vi "Trial v1.vi"(2 "error in (no error)":errorcluster, 3 "queue in":refnum<queue>, 4 "DDA":bool=TRUE) -> (0 "error out":errorcluster, 1 "queue out":refnum<queue>)   [LabVIEW 2017]
uses:
  SubVI/Global.vi
  <vilib>/Analysis/NI_AALPro.lvlib
  <vilib>/robotics/Kinematics/NI_Kinematics.lvlib
  Control/RPY.ctl
  Control/Damping.ctl
  <vilib>/Analysis/NI_AALBase.lvlib
  <vilib>/Analysis/baseanly.llb/Real Dot Product.vi
  <vilib>/Analysis/_algsub.llb/Real Vector Norm.vi
panel:
  out "R":dbl
  out "Rbar":dbl
  out "delta":dbl
  in  "Algorithm Parameter":T1={"lambda w"=0.0, "lambda theta"=0.0, "alpha w"=0.0, "alpha theta"=0.0, "alpha Rbar"=0.1}
  in  "n":i32=3
  in  "Reward Parameter":cluster{"C":dbl, "alpha":dbl}={"C"=100.0, "alpha"=1.0}
  in  "lower limit (RoM)":dbl=15.0
  in  "upper limit (RoM)":dbl=85.0
  in  "Time Target (s)":dbl=1.0
  in  "epsilon":dbl=0.1
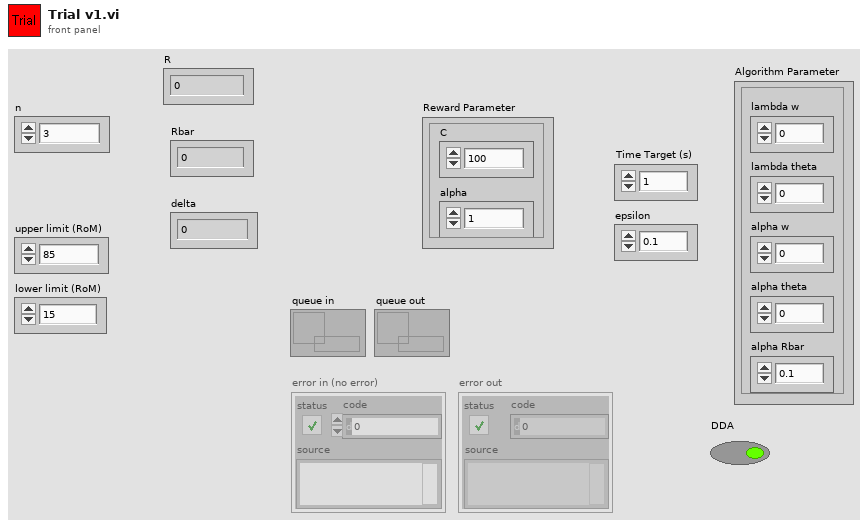
[diagram p1: front panel]
types:
  T1 = cluster{"lambda w":dbl, "lambda theta":dbl, "alpha w":dbl, "alpha theta":dbl, "alpha Rbar":dbl}
  T2 = typedef "Damping.ctl" = cluster{"Cx":dbl, "Cy":dbl, "Cz":dbl}
  T3 = typedef "RPY.ctl" = cluster{"roll":dbl, "pitch":dbl, "yaw":dbl}
  T4 = typedef "NI_Matrix.lvlib/RealMatrix.ctl" = dbl[][]
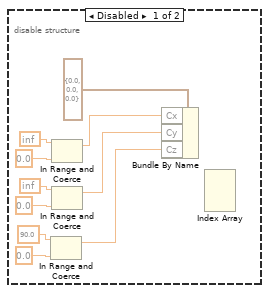
[diagram p2: hidden frame]
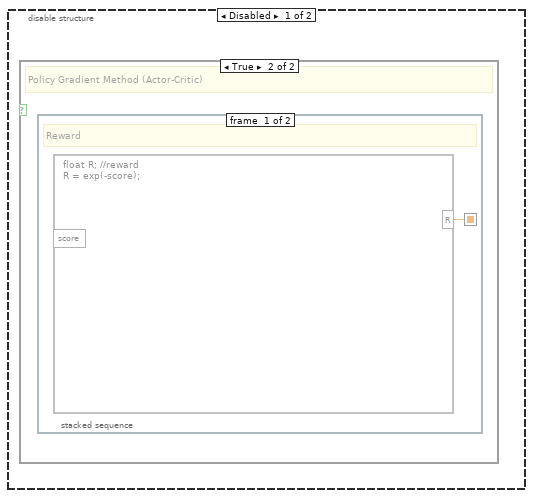
[diagram p3: hidden frame]
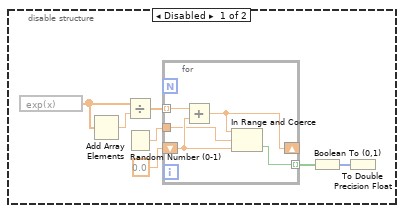
[diagram p6: hidden frame]
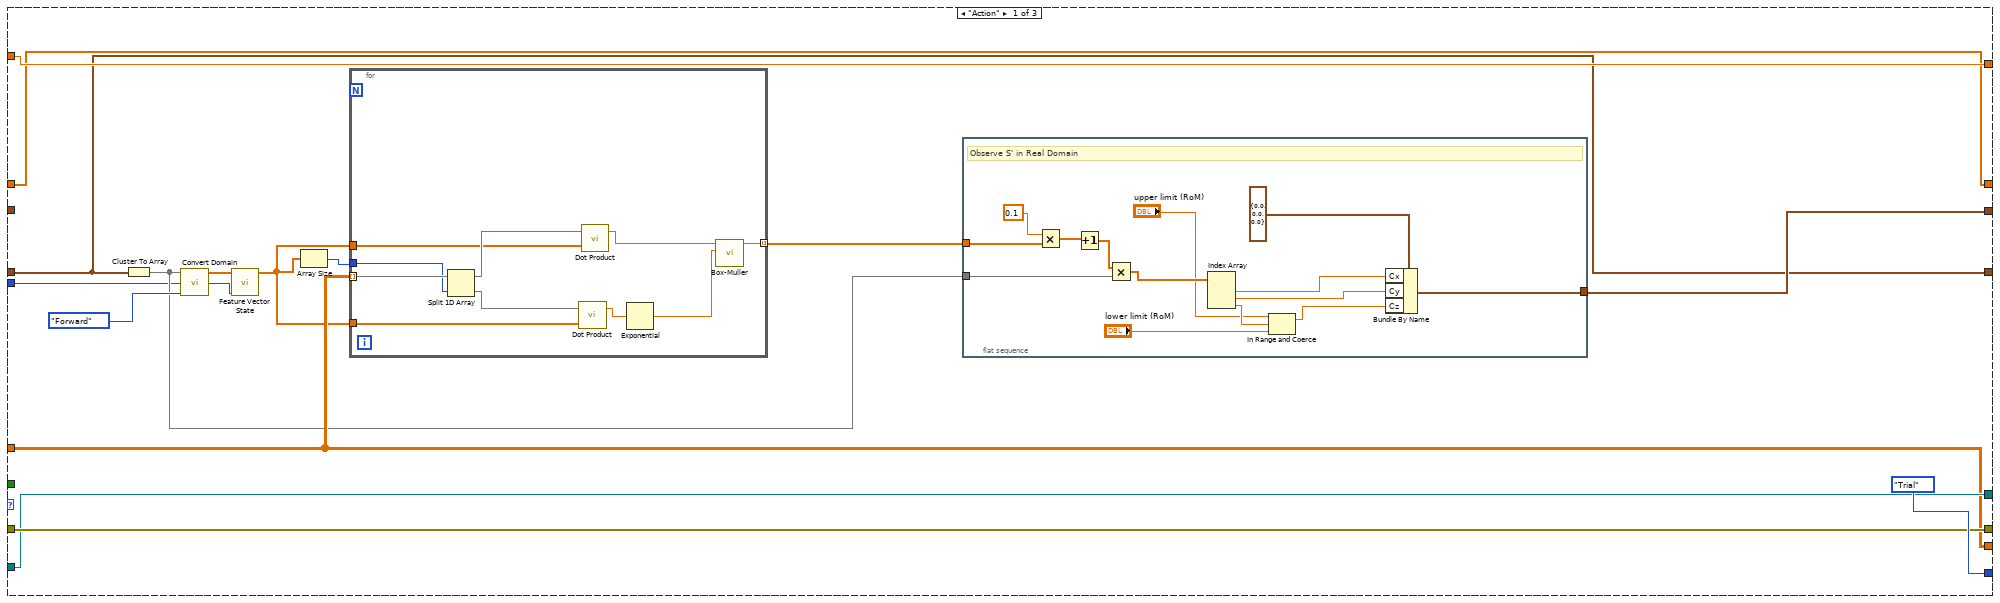
[diagram p7: hidden frame]
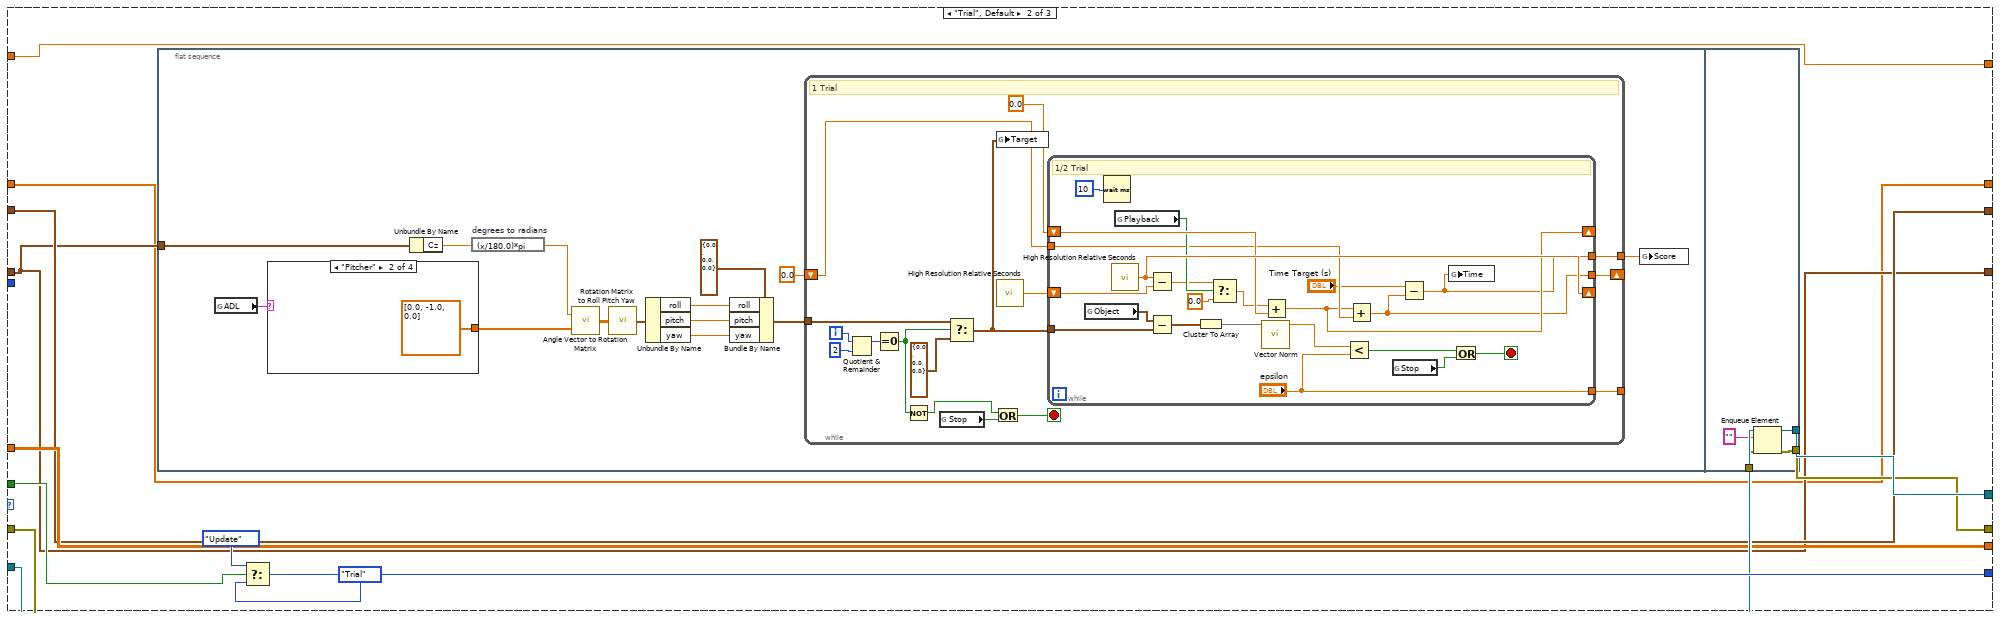
[diagram p8: hidden frame]
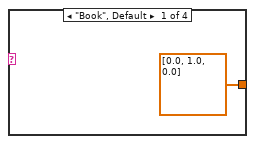
[diagram p9: hidden frame]
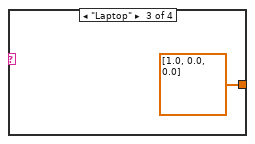
[diagram p10: hidden frame]
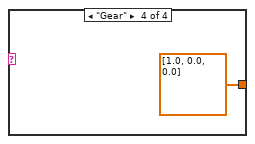
[diagram p11: hidden frame]
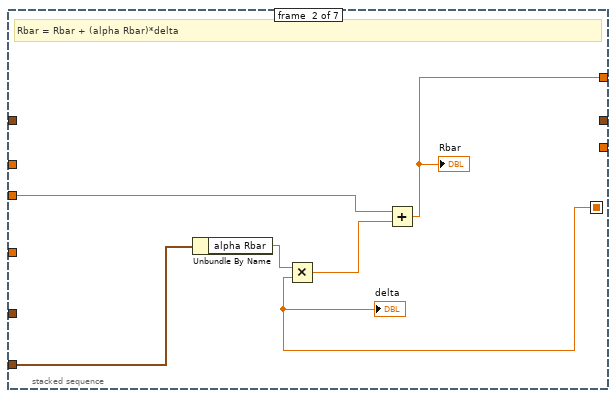
[diagram p12: hidden frame]
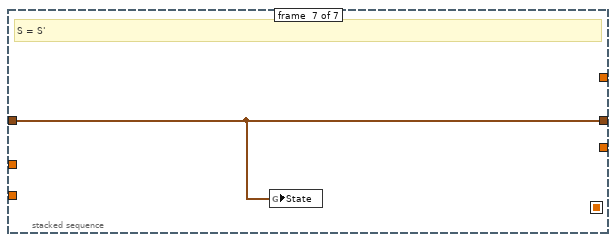
[diagram p17: hidden frame]
diagram:
  n1 = flat-sequence {
    tunnel: "error in (no error)" -> [w17]
    tunnel: "queue in" -> [w19]
    tunnel: "DDA" -> [w12]
    tunnel: [w18] -> w2
    tunnel: [w16] -> w1
    frame #0 {
      n2 = flat-sequence {
        tunnel: ["n"] -> w11
        tunnel: [w29] -> w10
        tunnel: [w28] -> w9
        tunnel: [w28] -> w8
        tunnel: [w26] -> w7
        tunnel: [w20] -> w6
        frame #0 {
          w29 = 0.0  # Rbar
          w22 = 0.0 ("element")
          w25 = dbl[] [0.0, 0.0, 0.0] ("array")
          n3 = call "Feature Vector State.vi"("n x(s)"="n", "state"=w25) -> ("x(s)"=w35:dbl[])  [unwired: 9 in]
          n4 = call "Feature Vector State.vi"("n x(s)"="n", "state"=w25) -> ("x(s)"=w33:dbl[])  [unwired: 9 in]
          n5 = call "Feature Vector State.vi"("n x(s)"="n", "state"=w25) -> ("x(s)"=w24:dbl[])  [unwired: 9 in]
          n6 = Array Size(array=w24) -> (size(s)=w23:i32)
          n7 = Array Size(array=w35) -> (size(s)=w34:i32)
          n8 = Array Size(array=w33) -> (size(s)=w32:i32)
          n9 = Initialize Array(w22, w23) -> (w20:dbl[])
          n10 = Initialize Array(w22, w34) -> (w31:dbl[])
          n11 = Initialize Array(w22, w32) -> (w30:dbl[])
          n12 = global read "Global.vi" "State"() -> (w28:T2)
          n13 = Build Array (concatenate)(w31, w30) -> (w27:dbl[])
          n14 = Build Array(w27, w27, w27) -> (w26:dbl[][])
        }
      }
      n15 = Select(t=enum16{"Action", "Trial", "Update"}."Action", s=w12, f=enum16{"Action", "Trial", "Update"}."Trial") -> (s? t:f=w13:enum16{"Action", "Trial", "Update"})
      n16 = while {
        shift-right: [w48] -> w18
        shift-left: w19 -> [w50]
        shift-right: [w47] -> w16
        shift-left: w17 -> [w49]
        shift-right: [w52] -> _
        shift-left: w13 -> [w53]
        tunnel: w12 -> [w51]
        tunnel: w11 -> [w46]
        shift-right: [w45] -> _
        shift-left: w7 -> [w44]
        shift-right: [w42] -> _
        shift-left: w10 -> [w43]
        shift-right: [w38] -> _
        shift-left: w9 -> [w40]
        shift-right: [w41] -> _
        shift-left: w8 -> [w39]
        shift-right: [w36] -> _
        shift-left: w6 -> [w37]
        stop <- w54 stop-if-true
        # "State Machine"
        n17 = case shown="\"Update\"" w53 {
          tunnel: [enum16{"Action", "Trial", "Update"}."Trial" w104 enum16{"Action", "Trial", "Update"}."Action"] -> w52
          tunnel: w51 -> [_ w106 _]
          tunnel: w50 -> [w65 w103 w182]
          tunnel: w49 -> [w66 w102 w183]
          tunnel: [w65 w101 w182] -> w48
          tunnel: [w66 w100 w183] -> w47
          tunnel: w46 -> [w57 _ w173]
          tunnel: [w64 w98 w184] -> w45
          tunnel: w44 -> [w64 w98 w184]
          tunnel: w43 -> [w60 w97 w175]
          tunnel: [w60 w97 w169] -> w42
          tunnel: w40 -> [w58 w95 w172]
          tunnel: [w59 w96 w171] -> w41
          tunnel: w39 -> [_ w96 w177]
          tunnel: [w58 w95 w171] -> w38
          tunnel: w37 -> [w55 w94 w174]
          tunnel: [w55 w94 w168] -> w36
          frame "Action" {
            n18 = Cluster To Array(cluster=w58) -> (array=w61:dbl[])
            n19 = call "Convert Domain.vi"("Direction"=enum16{"Forward", "Backward"}."Forward", "Real"=w61) -> ("Unit"=w67:dbl[])  [unwired: 9 in]
            n20 = call "Feature Vector State.vi"("n x(s)"=w57, "state"=w67) -> ("x(s)"=w56:dbl[])  [unwired: 9 in]
            n21 = Array Size(array=w56) -> (size(s)=w63:i32)
            n22 = for {
              tunnel: w64 -> [w93] mode=indexing
              tunnel: w56 -> [w90]
              tunnel: w56 -> [w89]
              tunnel: [w85] -> w62 mode=indexing
              tunnel: w63 -> [w84]
              n23 = Split 1D Array(array=w93, index=w84) -> (first subarray=w92:dbl[], second subarray=w91:dbl[])
              n24 = call-poly <vilib>:"Dot Product.vi"("Y Vector"=w89, "X Vector"=w91) -> ("X * Y"=w88:dbl)  [unwired: 1 out]
              n25 = call-poly <vilib>:"Dot Product.vi"("Y Vector"=w90, "X Vector"=w92) -> ("X * Y"=w87:dbl)  [unwired: 1 out]
              n26 = Exponential(1:w88) -> (0:w86:dbl)
              n27 = call "Box-Muller.vi"("sigma"=w86, "mu"=w87) -> ("x"=w85:dbl)  [unwired: 9 in]
            }
            n28 = flat-sequence {
              tunnel: w62 -> [w83]
              tunnel: w61 -> [w79]
              tunnel: [w70] -> w59
              frame #0 {
                # "Observe S' in Real Domain"
                n29 = Multiply(x=0.1, y=w83) -> (x*y=w81:dbl[])
                n30 = Increment(x=w81) -> (x+1=w80:dbl[])
                n31 = Multiply(x=w80, y=w79) -> (x*y=w75:dbl[])
                n32 = Index Array(array=w75) -> (element #1=w77:dbl, element #2=w76:dbl, element #3=w74:dbl)  [unwired: 3 in]
                n33 = In Range and Coerce(upper limit="upper limit (RoM)", x=w74, lower limit="lower limit (RoM)") -> (coerced(x)=w73:dbl)  [unwired: 1 out]
                n34 = Bundle By Name(cluster=T2 {"Cx"=0.0, "Cy"=0.0, "Cz"=0.0} ("State"), "Cx"=w77, "Cy"=w76, "Cz"=w73) -> (w70:T2)
              }
            }
          }
          frame "Trial", Default {
            n35 = flat-sequence {
              tunnel: w95 -> [w107]
              tunnel: w103 -> [w167]
              tunnel: w102 -> [w166]
              tunnel: [w165] -> w101
              tunnel: [w164] -> w100
              frame #0 {
                n36 = global read "Global.vi" "ADL"() -> (w111:string)
                n37 = case shown="\"Pitcher\"" w111 {
                  tunnel: [dbl[] [0.0, 1.0, 0.0] dbl[] [0.0, -1.0, 0.0] dbl[] [1.0, 0.0, 0.0] dbl[] [1.0, 0.0, 0.0]] -> w110
                  frame "Book", Default {
                  }
                  frame "Pitcher" {
                  }
                  frame "Laptop" {
                  }
                  frame "Gear" {
                  }
                }
                n38 = Unbundle By Name(w107) -> ("Cz"=w109:dbl)
                n39 = expression code="(x/180.0)*pi" "degrees to radians"(w109) -> (w112:dbl)
                n40 = call <vilib>:"Angle Vector to Rotation Matrix.vi"("vector"=w110, "angle"=w112) -> ("rotation matrix"=w115:T4)
                n41 = call <vilib>:"Rotation Matrix to Roll Pitch Yaw.vi"("rotation matrix"=w115) -> ("angles"=w116:cluster{"roll":dbl, "pitch":dbl, "yaw":dbl})
                n42 = Unbundle By Name(w116) -> ("roll"=w117:dbl, "pitch"=w118:dbl, "yaw"=w119:dbl)
                n43 = Bundle By Name(cluster=T3 {"roll"=0.0, "pitch"=0.0, "yaw"=0.0} ("Target"), "roll"=w117, "pitch"=w118, "yaw"=w119) -> (w113:T3)
                n44 = while {
                  tunnel: w113 -> [w135]
                  shift-right: [w127] -> _
                  shift-left: 0.0 -> [w128]
                  tunnel: [w126] -> _
                  tunnel: [w125] -> w108
                  i -> [w138]
                  stop <- w131 stop-if-true
                  # "1 Trial"
                  n45 = Quotient & Remainder(x=w138, y=2) -> (x-y*floor(x/y)=w136:i32)  [unwired: 1 out]
                  n46 = Equal To 0?(x=w136) -> (x = 0?=w130:bool)
                  n47 = Not(x=w130) -> (.not. x?=w129:bool)
                  n48 = global read "Global.vi" "Stop"() -> (w132:bool)
                  n49 = Select(t=w135, s=w130, f=T3 {"roll"=0.0, "pitch"=0.0, "yaw"=0.0} ("Target")) -> (s? t:f=w133:T3)
                  n50 = Or(x=w129, y=w132) -> (x .or. y?=w131:bool)
                  n51 = global write "Global.vi" "Target"(w133) -> ()
                  n52 = call <vilib>:"High Resolution Relative Seconds.vi"() -> ("relative seconds"=w140:dbl)
                  n53 = while {
                    tunnel: w133 -> [w147]
                    shift-right: [w153] -> _
                    shift-left: w140 -> [w154]
                    shift-right: [w145] -> _
                    shift-left: 0.0 -> [w152]
                    tunnel: w128 -> [w146]
                    tunnel: [w143] -> w127
                    tunnel: ["epsilon"] -> w126
                    tunnel: [w141] -> w125
                    stop <- w155 stop-if-true
                    # "1/2 Trial"
                    n54 = global read "Global.vi" "Object"() -> (w160:T3)
                    n55 = Wait (ms)(milliseconds to wait=u32 10) -> ()  [unwired: 1 out]
                    n56 = call <vilib>:"High Resolution Relative Seconds.vi"() -> ("relative seconds"=w153:dbl)
                    n57 = global read "Global.vi" "Playback"() -> (w151:bool)
                    n58 = Subtract(x=w153, y=w154) -> (x-y=w150:dbl)
                    n59 = Subtract(x=w160, y=w147) -> (x-y=w161:T3)
                    n60 = Cluster To Array(cluster=w161) -> (array=w162:dbl[])
                    n61 = Select(t=w150, s=w151, f=0.0) -> (s? t:f=w149:dbl)
                    n62 = call-poly <vilib>:"Vector Norm.vi"("Input Vector"=w162) -> ("norm"=w159:dbl)  [unwired: 9 in, 1 out]
                    n63 = Add(x=w149, y=w152) -> (x+y=w145:dbl)
                    n64 = Less?(x=w159, y="epsilon") -> (x < y?=w158:bool)
                    n65 = Add(x=w145, y=w146) -> (x+y=w143:dbl)
                    n66 = global read "Global.vi" "Stop"() -> (w157:bool)
                    n67 = Subtract(x="Time Target (s)", y=w143) -> (x-y=w141:dbl)
                    n68 = global write "Global.vi" "Time"(w141) -> ()
                    n69 = Or(x=w158, y=w157) -> (x .or. y?=w155:bool)
                  }
                }
                n70 = global write "Global.vi" "Score"(w108) -> ()
              }
              frame #1 {
                n71 = Enqueue Element(queue=w167, element="", error in (no error)=w166) -> (queue out=w165:refnum<queue>, error out=w164:errorcluster)  [unwired: 1 in, 1 out]
              }
            }
            n72 = Select(t=enum16{"Action", "Trial", "Update"}."Update", s=w106, f=enum16{"Action", "Trial", "Update"}."Trial") -> (s? t:f=w104:enum16{"Action", "Trial", "Update"})
          }
          frame "Update" {
            n73 = Unbundle By Name("Reward Parameter") -> ("C"=w179:dbl, "alpha"=w178:dbl)
            n74 = global read "Global.vi" "Score"() -> (w181:dbl)
            n75 = formula code="float R = C*exp(-alpha*abs(score));"("score"=w181, "C"=w179, "alpha"=w178) -> ("R"=w176:dbl)
            n76 = stacked-sequence {
              seq-local: [w186 _ _ _ _ _ _] -> [_ w202 _ _ _ _ _]
              tunnel: [_ _ _ _ _ _ w207] -> w171
              tunnel: w177 -> [w195 _ _ _ _ _ w207]
              tunnel: w176 -> [w199 _ _ _ _ _ _]
              tunnel: w175 -> [w198 w205 _ _ _ _ _]
              tunnel: w174 -> [w196 _ _ _ w206 _ _]
              tunnel: w173 -> [w189 _ _ _ _ _ _]
              tunnel: w172 -> [w194 _ _ _ _ _ _]
              tunnel: "Algorithm Parameter" -> [_ w204 _ _ _ _ _]
              tunnel: [_ w200 _ _ _ _ _] -> w169
              tunnel: [_ _ _ _ w206 _ _] -> w168
              frame #0 {
                # "delta = R - Rbar + vhat(S', w) - vhat(S,w)"
                n77 = Subtract(x=w195, y=w194) -> (x-y=w193:T2)
                n78 = Cluster To Array(cluster=w193) -> (array=w192:dbl[])
                n79 = Subtract(x=w199, y=w198) -> (x-y=w197:dbl)
                n80 = call "Convert Domain.vi"("Direction"=enum16{"Forward", "Backward"}."Forward", "Real"=w192) -> ("Unit"=w190:dbl[])  [unwired: 9 in]
                n81 = call "Feature Vector State.vi"("n x(s)"=w189, "state"=w190) -> ("x(s)"=w188:dbl[])  [unwired: 9 in]
                n82 = call-poly <vilib>:"Dot Product.vi"("Y Vector"=w188, "X Vector"=w196) -> ("X * Y"=w187:dbl)  [unwired: 1 out]
                n83 = Add(x=w197, y=w187) -> (x+y=w186:dbl)
                "R" <- w199
              }
              frame #1 {
                # "Rbar = Rbar + (alpha Rbar)*delta"
                n84 = Unbundle By Name(w204) -> ("alpha Rbar"=w203:dbl)
                n85 = Multiply(x=w203, y=w202) -> (x*y=w201:dbl)
                n86 = Add(x=w205, y=w201) -> (x+y=w200:dbl)
                "Rbar" <- w200
                "delta" <- w202
              }
              frame #2 {
                # "zw = (lamda w)*zw + del vhat(S, w)"
              }
              frame #3 {
                # "ztheta = (lambda theta)*ztheta + del ln(pi(A| S, theta))"
              }
              frame #4 {
                # "w = w + (alpha w)*delta*zw"
              }
              frame #5 {
                # "theta = theta + (alpha theta)*delta*ztheta"
              }
              frame #6 {
                # "S = S'"
                n87 = global write "Global.vi" "State"(w207) -> ()
              }
            }
          }
        }
        n88 = global read "Global.vi" "Stop"() -> (w54:bool)
      }
    }
  }
  n89 = disable-structure shown="Enabled" {
    frame Disabled {
      n90 = In Range and Coerce(upper limit=90.0, lower limit=0.0) -> (coerced(x)=w217:dbl)  [unwired: 1 in, 1 out]
      n91 = In Range and Coerce(upper limit=inf, lower limit=0.0) -> (coerced(x)=w215:dbl)  [unwired: 1 in, 1 out]
      n92 = In Range and Coerce(upper limit=inf, lower limit=0.0) -> (coerced(x)=w216:dbl)  [unwired: 1 in, 1 out]
      n93 = Bundle By Name(cluster=T2 {"Cx"=0.0, "Cy"=0.0, "Cz"=0.0} ("State"), "Cx"=w215, "Cy"=w216, "Cz"=w217) -> ()  [unwired: 1 out]
      n94 = Index Array() -> ()  [unwired: 4 in, 3 out]
    }
    frame Enabled {
    }
  }
  n95 = disable-structure shown="Enabled" {
    frame Disabled {
      n96 = expression code="exp(x)"() -> (w220:dbl[])  [unwired: 1 in]
      n97 = Add Array Elements(numeric array=w220) -> (sum=w221:dbl)
      n98 = Divide(x=w220, y=w221) -> (x/y=w218:dbl[])
      n99 = Random Number (0-1)() -> (number: 0 to 1=w222:dbl)
      n100 = for {
        shift-right: [w228] -> _
        shift-left: 0.0 -> [w229]
        tunnel: w222 -> [w227]
        tunnel: [w226] -> w223 mode=indexing
        tunnel: w218 -> [w225] mode=indexing
        n101 = Add(x=w225, y=w229) -> (x+y=w228:dbl)
        n102 = In Range and Coerce(upper limit=w228, x=w227, lower limit=w229) -> (In Range?=w226:bool)  [unwired: 1 out]
      }
      n103 = Boolean To (0,1)(Boolean=w223) -> (0, 1=w224:i16[])
      n104 = To Double Precision Float(number=w224) -> ()  [unwired: 1 out]
    }
    frame Enabled {
    }
  }
  n105 = disable-structure shown="Enabled" {
    frame Disabled {
      n106 = case shown="True" {
        selector: _ -> [_ _]
        frame False {
        }
        frame True {
          # "Policy Gradient Method (Actor-Critic)"
          n107 = stacked-sequence {
            seq-local: [w230 _] -> [_ _]
            frame #0 {
              # "Reward"
              n108 = formula code="float R; //reward\nR = exp(-score);"() -> ("R"=w230:dbl)  [unwired: 1 in]
            }
            frame #1 {
            }
          }
        }
      }
    }
    frame Enabled {
    }
  }
  "error out" <- w1
  "queue out" <- w2
